vi "Auton Commands.vi"(9 "Distance":dbl=120.0, 10 "Task":string) -> ()   [LabVIEW 2015]
uses:
  <vilib>/Rock Robotics/Network Tables/NT Read Number.vi
  <vilib>/Rock Robotics/WPI/Utilities/WPI_GetSetVariantRefNum.vi
  <vilib>/addons/control/pid/pid.llb/PID (DBL).vi
  <vilib>/Rock Robotics/Network Tables/NT Write Number.vi
  <vilib>/addons/control/pid/NI_PID_pid.lvlib
  navX Library v2/navX Library v2.lvlib
panel:
  out "Yaw":dbl(graph)
  out "E1 Rate":dbl
  out "E2 Rate":dbl
  in  "Yaw Gains":T1={"proportional gain (Kc)"=0.2, "integral time (Ti, min)"=0.0, "derivative time (Td, min)"=0.0} {"derivative time (Td, min)" format="%.3f"; "integral time (Ti, min)" format="%.3f"; "proportional gain (Kc)" format="%.3f"}
  in  "Speed Gains":T1={"proportional gain (Kc)"=0.65, "integral time (Ti, min)"=0.001, "derivative time (Td, min)"=0.001} {"derivative time (Td, min)" format="%.3f"; "integral time (Ti, min)" format="%.3f"; "proportional gain (Kc)" format="%.3f"}
  in  "Single Turn Gains":T1={"proportional gain (Kc)"=0.12, "integral time (Ti, min)"=0.0, "derivative time (Td, min)"=0.0} {"derivative time (Td, min)" format="%.3f"; "integral time (Ti, min)" format="%.3f"; "proportional gain (Kc)" format="%.3f"}
  out "Right Motor Speed":dbl(graph)
  out "Left Motor Speed":dbl(graph)
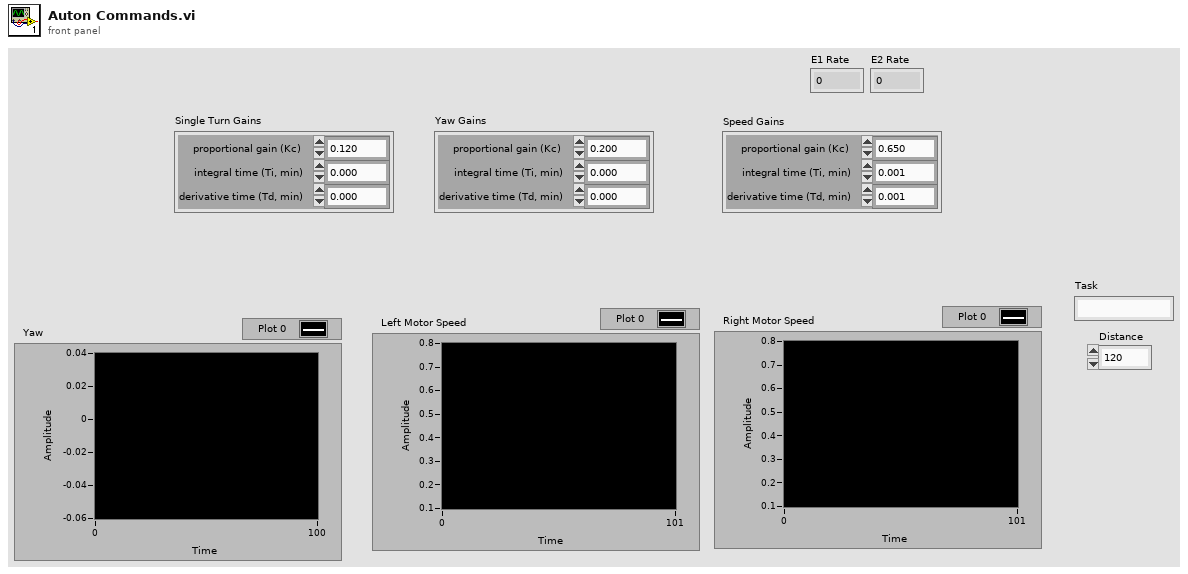
[diagram p1: front panel]
types:
  T1 = cluster{"proportional gain (Kc)":dbl, "integral time (Ti, min)":dbl, "derivative time (Td, min)":dbl}
  T2 = typedef "navX Library v2.lvlib/Z900_navX_DeviceTypeDef.ctl" = cluster{"Interface":cluster{"Protocol":T3, "Update Rate (4Hz-60Hz)":u8, "navX Open TypeDef":variant}, "Notify Packet":refnum<notifier>, "Loop VI Refnum":refnum<vi>, "Ready to Close Occurrence Refnum":refnum<k4>}
  T3 = typedef "navX Library v2.lvlib/Z900_navX_ProtocolTypeDef.ctl" = enum16{"SERIAL", "I2C", "SPI"}
  T4 = typedef "WPI_EncoderDevRef.ctl" = cluster{"DevStatus":errorcluster, "EncoderIndex":T5, "CounterIndex":T6, "DistancePerCount":dbl, "Decoding Type":T7}
  T5 = typedef "FPGA_EncoderIdx.ctl" = enum8{"Enc 0", "Enc 1", "Enc 2", "Enc 3", "Enc 4", "Enc 5", "Enc 6", "Enc 7", "Invalid"}
  T6 = typedef "FPGA_CounterCtrSystemIndex.ctl" = enum8{"Ctr 0", "Ctr 1", "Ctr 2", "Ctr 3", "Ctr 4", "Ctr 5", "Ctr 6", "Ctr 7", "Invalid"}
  T7 = typedef "WPI_EncoderType.ctl" = enum16{"1x", "2x", "4x"}
  T8 = cluster{"Yaw":dbl, "Roll":dbl, "Pitch":dbl, "Heading":dbl, "Fused Heading":dbl}
  T9 = typedef "WPI_RobotDriveDevRef.ctl" = cluster{"DevStatus":errorcluster, "Motors[]":T10[], "Square Inputs":bool, "Max Output":dbl}
  T10 = typedef "WPI_MotorControlDeviceRef.ctl" = cluster{"DeviceStatus":errorcluster, "Type":T11, "PWM":cluster{"PWM Channel":T12, "DeadBand":T13}, "CAN":cluster{"Device Number":u8, "Control Mode":T14, "Semaphore":T15, "Max Vout":dbl, "TalonSRX Control Mode":T16}, "Invert":bool}
  T11 = typedef "WPI_MotorControlType.ctl" = enum16{"PWM", "CAN", "CANTalonSRX"}
  T12 = typedef "FPGA_DIOPWMChannel.ctl" = enum8{"PWM 0", "PWM 1", "PWM 2", "PWM 3", "PWM 4", "PWM 5", "PWM 6", "PWM 7", "PWM 8", "PWM 9", "PWM MXP 0", "PWM MXP 1", "PWM MXP 2", "PWM MXP 3", "PWM MXP 4", "PWM MXP 5", "PWM MXP 6", "PWM MXP 7", "PWM MXP 8", "PWM MXP 9", "Invalid"}
  T13 = typedef "WPI_PWMDeadband.ctl" = cluster{"Name":string, "maxPositivePwm":i32, "minPositivePwm":i32, "centerPwm":i32, "maxNegativePwm":i32, "minNegativePwm":i32, "angularRange":u16}
  T14 = typedef "WPI_CANJaguar_ControlMode.ctl" = enum8{"Percent VBus", "Current", "Speed", "Position", "Voltage"}
  T15 = typedef "Semaphore RefNum" = refnum<k1>
  T16 = typedef "WPI_CANTalonSRX_APIControlMode.ctl" = enum8{"Percent VBus", "Speed", "Position", "Slave", "Unchanged / Invalid", "Voltage Compensation", "Current", "Motion Profile"}
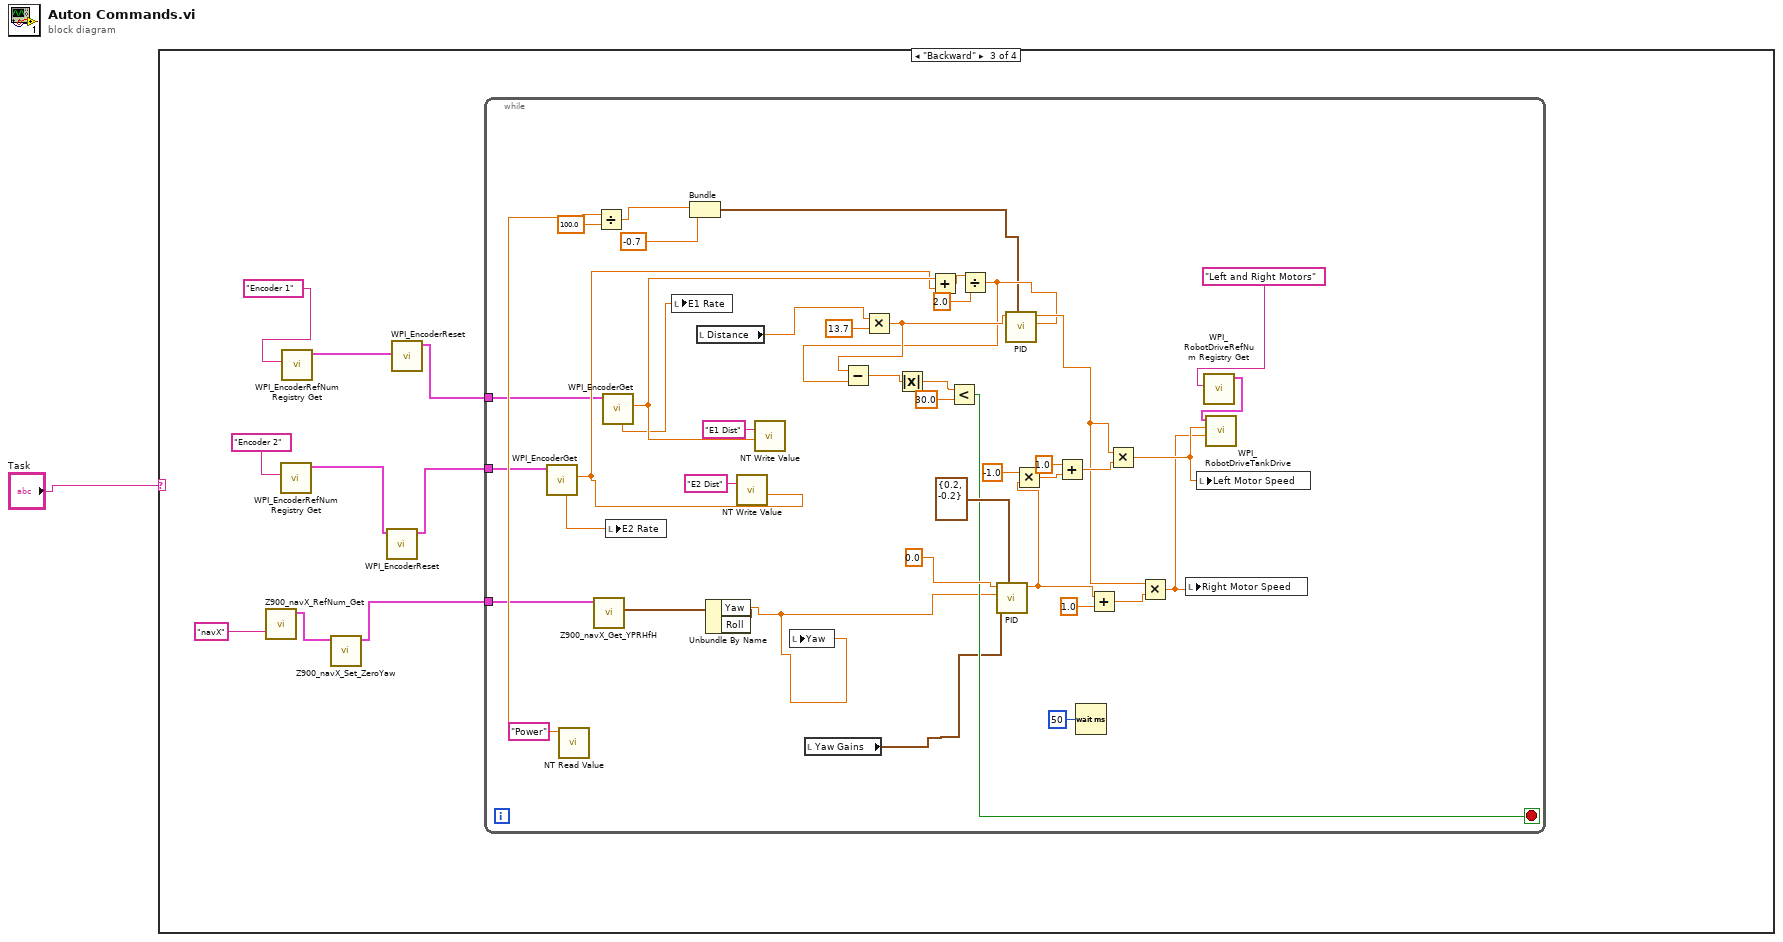
[diagram p0: block diagram]
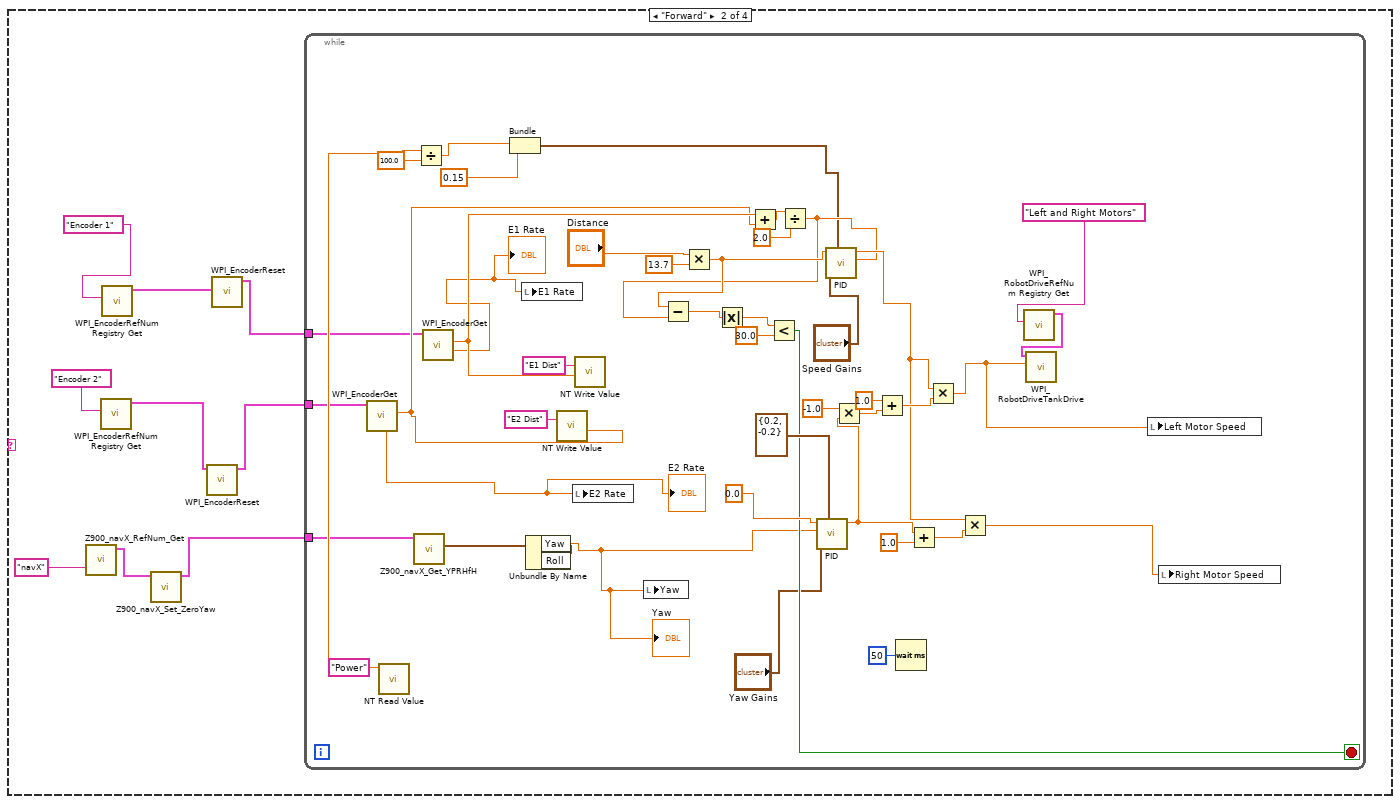
[diagram p3: hidden frame]
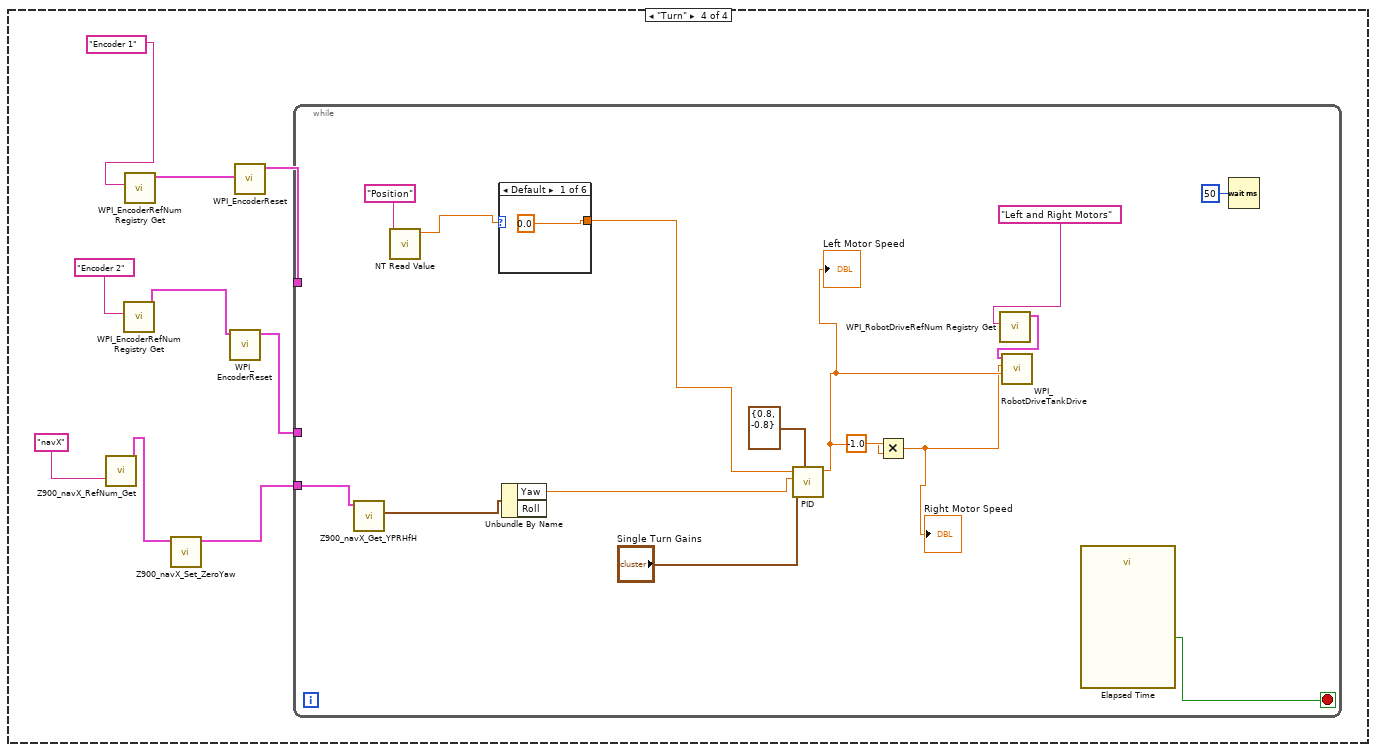
[diagram p4: hidden frame]
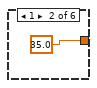
[diagram p5: hidden frame]
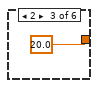
[diagram p6: hidden frame]
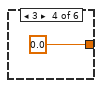
[diagram p7: hidden frame]
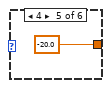
[diagram p8: hidden frame]
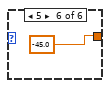
[diagram p9: hidden frame]
diagram:
  n1 = case shown="\"Backward\"" "Task" {
    frame Default {
    }
    frame "Forward" {
      n2 = call "Z900_navX_RefNum_Get.vi"("refnum name"="navX") -> ("navX Device"=w10:T2)  [unwired: 9 in, 1 out]
      n3 = call <vilib>:"WPI_EncoderRefNum Registry Get.vi"("refnum name"="Encoder 2") -> ("EncoderDevRef"=w9:T4)  [unwired: 9 in, 1 out]
      n4 = call <vilib>:"WPI_EncoderRefNum Registry Get.vi"("refnum name"="Encoder 1") -> ("EncoderDevRef"=w8:T4)  [unwired: 9 in, 1 out]
      n5 = call "Z900_navX_Set_ZeroYaw.vi"("navX Device"=w10) -> ("navX Device"=w2:T2)  [unwired: 9 in, 1 out]
      n6 = call <vilib>:"WPI_EncoderReset.vi"("EncoderDevRef"=w9) -> ("EncoderDevRef"=w3:T4)  [unwired: 9 in, 1 out]
      n7 = call <vilib>:"WPI_EncoderReset.vi"("EncoderDevRef"=w8) -> ("EncoderDevRef"=w4:T4)  [unwired: 9 in, 1 out]
      n8 = while {
        tunnel: w4 -> [w21]
        tunnel: w3 -> [w20]
        tunnel: w2 -> [w19]
        stop <- w27 stop-if-true
        n9 = call <vilib>:"WPI_EncoderGet.vi"("EncoderDevRef"=w20) -> ("Distance"=w33:dbl, "Rate"=w18:dbl)  [unwired: 5 in, 4 out]
        "E2 Rate" <- w18
        n10 = call-poly <vilib>:"NT Read Value.vi"("Name"="Power") -> ("Numeric"=w26:dbl)  [unwired: 9 in, 1 out]
        n11 = call "Z900_navX_Get_YPRHfH.vi"("navX Device"=w19) -> ("YRPHfH"=w49:T8)  [unwired: 7 in, 3 out]
        n12 = Divide(x=w26, y=100.0) -> (x/y=w24:dbl)
        n13 = call <vilib>:"WPI_EncoderGet.vi"("EncoderDevRef"=w21) -> ("Distance"=w34:dbl, "Rate"=w17:dbl)  [unwired: 5 in, 4 out]
        "E1 Rate" <- w17
        n14 = Bundle(w24, "output low"=0.15) -> (w22:cluster{dbl, "output low":dbl})  [unwired: 1 in]
        n15 = local write "E1 Rate"(w17) -> ()
        n16 = Unbundle By Name(w49) -> ("Yaw"=w14:dbl)  [unwired: 1 out]
        "Yaw" <- w14
        n17 = call-poly <vilib>:"NT Write Value.vi"("Numeric"=w33, "Name"="E2 Dist") -> ()  [unwired: 9 in, 1 out]
        n18 = local write "E2 Rate"(w18) -> ()
        n19 = call-poly <vilib>:"NT Write Value.vi"("Numeric"=w34, "Name"="E1 Dist") -> ()  [unwired: 9 in, 1 out]
        n20 = local write "Yaw"(w14) -> ()
        n21 = Multiply(x="Distance", y=13.7) -> (x*y=w32:dbl)
        n22 = Add(x=w34, y=w33) -> (x+y=w48:dbl)
        n23 = Divide(x=w48, y=2.0) -> (x/y=w31:dbl)
        n24 = Subtract(x=w32, y=w31) -> (x-y=w30:dbl)
        n25 = Absolute Value(x=w30) -> (abs(x)=w29:dbl)
        n26 = Less?(x=w29, y=30.0) -> (x < y?=w27:bool)
        n27 = call-poly <vilib>:"PID.vi"("output range"=cluster{"output high":dbl, "output low":dbl} {"output high"=0.2, "output low"=-0.2}, "PID gains"="Yaw Gains", "process variable"=w14, "setpoint"=0.0) -> ("output"=w41:dbl)  [unwired: 6 in, 1 out]
        n28 = call-poly <vilib>:"PID.vi"("output range"=w22, "PID gains"="Speed Gains", "process variable"=w31, "setpoint"=w32) -> ("output"=w38:dbl)  [unwired: 6 in, 1 out]
        n29 = Multiply(x=-1.0, y=w41) -> (x*y=w42:dbl)
        n30 = Add(x=1.0, y=w42) -> (x+y=w43:dbl)
        n31 = Wait (ms)(milliseconds to wait=u32 50) -> ()  [unwired: 1 out]
        n32 = Add(x=w41, y=1.0) -> (x+y=w44:dbl)
        n33 = Multiply(x=w38, y=w43) -> (x*y=w36:dbl)
        n34 = Multiply(x=w38, y=w44) -> (x*y=w11:dbl)
        n35 = call <vilib>:"WPI_RobotDriveRefNum Registry Get.vi"("refnum name"="Left and Right Motors") -> ("RobotDriveDevRef"=w51:T9)  [unwired: 9 in, 1 out]
        n36 = call <vilib>:"WPI_RobotDriveTankDrive.vi"("Left axis value"=w36, "RobotDriveDevRef"=w51) -> ()  [unwired: 7 in, 3 out]
        n37 = local write "Left Motor Speed"(w36) -> ()
        n38 = local write "Right Motor Speed"(w11) -> ()
      }
    }
    frame "Backward" {
      n39 = call "Z900_navX_RefNum_Get.vi"("refnum name"="navX") -> ("navX Device"=w63:T2)  [unwired: 9 in, 1 out]
      n40 = call <vilib>:"WPI_EncoderRefNum Registry Get.vi"("refnum name"="Encoder 2") -> ("EncoderDevRef"=w62:T4)  [unwired: 9 in, 1 out]
      n41 = call <vilib>:"WPI_EncoderRefNum Registry Get.vi"("refnum name"="Encoder 1") -> ("EncoderDevRef"=w61:T4)  [unwired: 9 in, 1 out]
      n42 = call "Z900_navX_Set_ZeroYaw.vi"("navX Device"=w63) -> ("navX Device"=w55:T2)  [unwired: 9 in, 1 out]
      n43 = call <vilib>:"WPI_EncoderReset.vi"("EncoderDevRef"=w62) -> ("EncoderDevRef"=w56:T4)  [unwired: 9 in, 1 out]
      n44 = call <vilib>:"WPI_EncoderReset.vi"("EncoderDevRef"=w61) -> ("EncoderDevRef"=w57:T4)  [unwired: 9 in, 1 out]
      n45 = while {
        tunnel: w57 -> [w74]
        tunnel: w56 -> [w73]
        tunnel: w55 -> [w72]
        stop <- w80 stop-if-true
        n46 = call <vilib>:"WPI_EncoderGet.vi"("EncoderDevRef"=w73) -> ("Distance"=w86:dbl, "Rate"=w68:dbl)  [unwired: 5 in, 4 out]
        n47 = call-poly <vilib>:"NT Read Value.vi"("Name"="Power") -> ("Numeric"=w79:dbl)  [unwired: 9 in, 1 out]
        n48 = call "Z900_navX_Get_YPRHfH.vi"("navX Device"=w72) -> ("YRPHfH"=w101:T8)  [unwired: 7 in, 3 out]
        n49 = Divide(x=w79, y=100.0) -> (x/y=w77:dbl)
        n50 = call <vilib>:"WPI_EncoderGet.vi"("EncoderDevRef"=w74) -> ("Distance"=w87:dbl, "Rate"=w67:dbl)  [unwired: 5 in, 4 out]
        n51 = local write "E2 Rate"(w68) -> ()
        n52 = local write "E1 Rate"(w67) -> ()
        n53 = Bundle(w77, "output low"=-0.7) -> (w75:cluster{dbl, "output low":dbl})  [unwired: 1 in]
        n54 = local read "Distance"() -> (w66:dbl)
        n55 = Unbundle By Name(w101) -> ("Yaw"=w70:dbl)  [unwired: 1 out]
        n56 = call-poly <vilib>:"NT Write Value.vi"("Numeric"=w86, "Name"="E2 Dist") -> ()  [unwired: 9 in, 1 out]
        n57 = call-poly <vilib>:"NT Write Value.vi"("Numeric"=w87, "Name"="E1 Dist") -> ()  [unwired: 9 in, 1 out]
        n58 = local write "Yaw"(w70) -> ()
        n59 = local read "Yaw Gains"() -> (w69:T1)
        n60 = Multiply(x=w66, y=13.7) -> (x*y=w85:dbl)
        n61 = Add(x=w87, y=w86) -> (x+y=w100:dbl)
        n62 = Divide(x=w100, y=2.0) -> (x/y=w84:dbl)
        n63 = Subtract(x=w85, y=w84) -> (x-y=w83:dbl)
        n64 = Absolute Value(x=w83) -> (abs(x)=w82:dbl)
        n65 = Less?(x=w82, y=30.0) -> (x < y?=w80:bool)
        n66 = call-poly <vilib>:"PID.vi"("output range"=cluster{"output high":dbl, "output low":dbl} {"output high"=0.2, "output low"=-0.2}, "PID gains"=w69, "process variable"=w70, "setpoint"=0.0) -> ("output"=w93:dbl)  [unwired: 6 in, 1 out]
        n67 = call-poly <vilib>:"PID.vi"("output range"=w75, "process variable"=w84, "setpoint"=w85) -> ("output"=w90:dbl)  [unwired: 7 in, 1 out]
        n68 = Multiply(x=-1.0, y=w93) -> (x*y=w94:dbl)
        n69 = Add(x=1.0, y=w94) -> (x+y=w95:dbl)
        n70 = Wait (ms)(milliseconds to wait=u32 50) -> ()  [unwired: 1 out]
        n71 = Add(x=w93, y=1.0) -> (x+y=w96:dbl)
        n72 = Multiply(x=w90, y=w95) -> (x*y=w65:dbl)
        n73 = Multiply(x=w90, y=w96) -> (x*y=w64:dbl)
        n74 = local write "Right Motor Speed"(w64) -> ()
        n75 = local write "Left Motor Speed"(w65) -> ()
        n76 = call <vilib>:"WPI_RobotDriveRefNum Registry Get.vi"("refnum name"="Left and Right Motors") -> ("RobotDriveDevRef"=w103:T9)  [unwired: 9 in, 1 out]
        n77 = call <vilib>:"WPI_RobotDriveTankDrive.vi"("Right axis value"=w64, "Left axis value"=w65, "RobotDriveDevRef"=w103) -> ()  [unwired: 6 in, 3 out]
      }
    }
    frame "Turn" {
      n78 = call "Z900_navX_RefNum_Get.vi"("refnum name"="navX") -> ("navX Device"=w108:T2)  [unwired: 9 in, 1 out]
      n79 = call <vilib>:"WPI_EncoderRefNum Registry Get.vi"("refnum name"="Encoder 2") -> ("EncoderDevRef"=w110:T4)  [unwired: 9 in, 1 out]
      n80 = call <vilib>:"WPI_EncoderRefNum Registry Get.vi"("refnum name"="Encoder 1") -> ("EncoderDevRef"=w112:T4)  [unwired: 9 in, 1 out]
      n81 = call "Z900_navX_Set_ZeroYaw.vi"("navX Device"=w108) -> ("navX Device"=w107:T2)  [unwired: 9 in, 1 out]
      n82 = call <vilib>:"WPI_EncoderReset.vi"("EncoderDevRef"=w110) -> ("EncoderDevRef"=w109:T4)  [unwired: 9 in, 1 out]
      n83 = call <vilib>:"WPI_EncoderReset.vi"("EncoderDevRef"=w112) -> ("EncoderDevRef"=w111:T4)  [unwired: 9 in, 1 out]
      n84 = while {
        tunnel: w111 -> [_]
        tunnel: w109 -> [_]
        tunnel: w107 -> [w126]
        stop <- w122 stop-if-true
        n85 = call "Z900_navX_Get_YPRHfH.vi"("navX Device"=w126) -> ("YRPHfH"=w125:T8)  [unwired: 7 in, 3 out]
        n86 = call-poly <vilib>:"NT Read Value.vi"("Name"="Position") -> ("Numeric"=w119:dbl)  [unwired: 9 in, 1 out]
        n87 = case shown="Default" w119 {
          tunnel: [0.0 35.0 20.0 0.0 -20.0 -45.0] -> w120
          frame Default {
          }
          frame 1 {
          }
          frame 2 {
          }
          frame 3 {
          }
          frame 4 {
          }
          frame 5 {
          }
        }
        n88 = Unbundle By Name(w125) -> ("Yaw"=w123:dbl)  [unwired: 1 out]
        n89 = call-poly <vilib>:"PID.vi"("output range"=cluster{"output high":dbl, "output low":dbl} {"output high"=0.8, "output low"=-0.8}, "PID gains"="Single Turn Gains", "process variable"=w123, "setpoint"=w120) -> ("output"=w117:dbl)  [unwired: 6 in, 1 out]
        "Left Motor Speed" <- w117
        n90 = Multiply(x=-1.0, y=w117) -> (x*y=w116:dbl)
        "Right Motor Speed" <- w116
        n91 = call <vilib>:"WPI_RobotDriveRefNum Registry Get.vi"("refnum name"="Left and Right Motors") -> ("RobotDriveDevRef"=w129:T9)  [unwired: 9 in, 1 out]
        n92 = call <vilib>:"WPI_RobotDriveTankDrive.vi"("Right axis value"=w117, "Left axis value"=w116, "RobotDriveDevRef"=w129) -> ()  [unwired: 6 in, 3 out]
        n93 = call "Elapsed Time"() -> ("Time has Elapsed"=w122:bool)  [unwired: 12 in, 7 out]
        n94 = Wait (ms)(milliseconds to wait=u32 50) -> ()  [unwired: 1 out]
      }
    }
  }
